vi "WaitForCommand.vi"(8 "error in (no error)":errorcluster, 11 "RobotSubsystem in":refnum<class "RobotSubsystem.lvclass">) -> (0 "error out":errorcluster, 3 "RobotSubsystem out":refnum<class "RobotSubsystem.lvclass">)   [LabVIEW 2017, in "RobotSubsystem.lvclass"]
uses:
  RobotSubsystem.lvclass
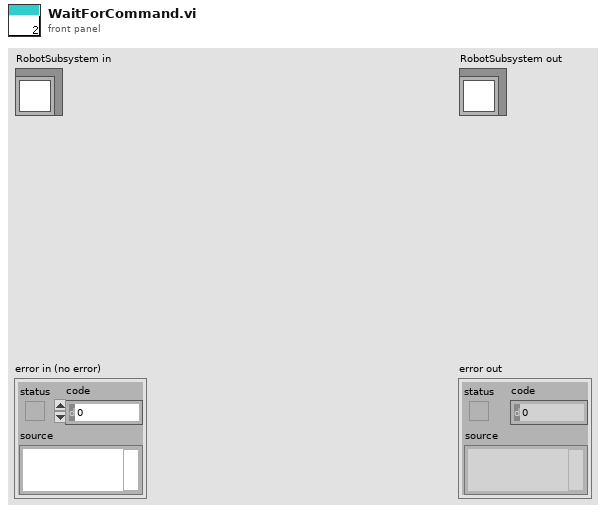
[diagram p1: front panel]
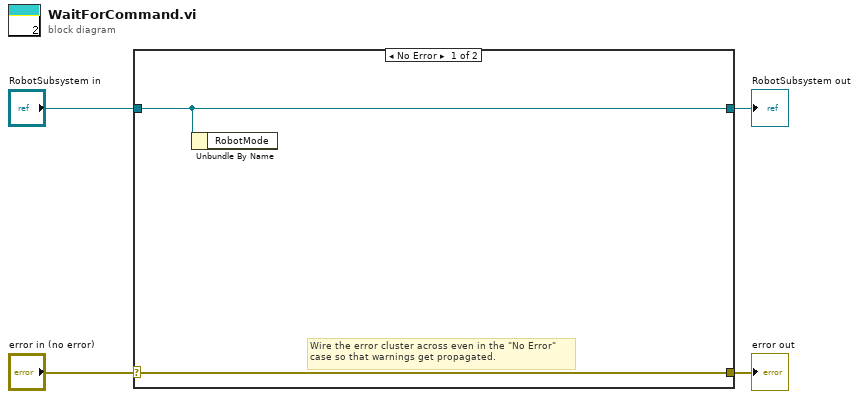
[diagram p0: block diagram]
diagram:
  n1 = case shown="No Error" "error in (no error)" {
    selector: "error in (no error)" -> [w6 w8]
    tunnel: [w6 w8] -> w3
    tunnel: [w5 w7] -> w1
    tunnel: "RobotSubsystem in" -> [w5 w7]
    frame No Error {
      # "Wire the error cluster across even in the \"No Error\"\ncase so that warnings get propagated."
      n2 = Unbundle By Name(w5) -> ()  [unwired: 1 out]
    }
    frame Error {
    }
  }
  "error out" <- w3
  "RobotSubsystem out" <- w1
